vi "JKISM++ Convert Data to HexStr.vi"(2 "Variant":variant) -> (7 "HEX String (0-9,A-F)":string)   [LabVIEW 2014, in "JKI State Machine++.lvlib"]
doc: "Convert complex argument(variant) to hex string, which could be safely used as state argument without broking the string queue logic.\n\n<b>Inputs:</b>\n - <b>Variant</b>: Complex data in variant format.\n\n<b>Outputs:</b>\n - <b>HEX String (0-9,A-F)</b>: Hex String, which contains no invisible string following JKISM's rule"
uses:
  JKI State Machine++.lvlib
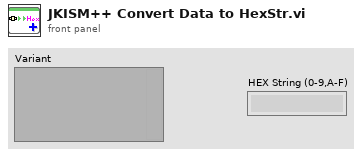
[diagram p1: front panel]
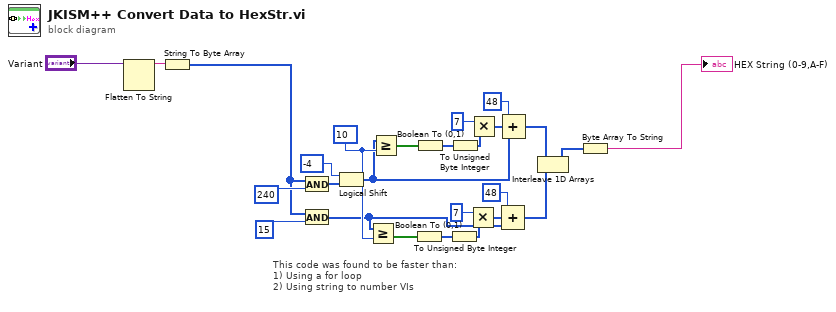
[diagram p0: block diagram]
diagram:
  w20 = u8 10
  # "This code was found to be faster than:\n1) Using a for loop\n2) Using string to number VIs"
  n1 = Flatten To String(anything="Variant") -> (data string=w25:string)  [unwired: 3 in, 2 out]
  n2 = String To Byte Array(string=w25) -> (unsigned byte array=w1:u8[])
  n3 = And(x=w1, y=u8 240) -> (x .and. y?=w22:u8[])
  n4 = And(x=w1, y=u8 15) -> (x .and. y?=w4:u8[])
  n5 = Logical Shift(y=i8 -4, x=w22) -> (x << y=w13:u8[])
  n6 = Greater Or Equal?(x=w4, y=w20) -> (x >= y?=w5:bool[])
  n7 = Greater Or Equal?(x=w13, y=w20) -> (x >= y?=w14:bool[])
  n8 = Boolean To (0,1)(Boolean=w5) -> (0, 1=w7:i16[])
  n9 = Boolean To (0,1)(Boolean=w14) -> (0, 1=w19:i16[])
  n10 = To Unsigned Byte Integer(number=w7) -> (unsigned 8bit integer=w8:u8[])
  n11 = To Unsigned Byte Integer(number=w19) -> (unsigned 8bit integer=w18:u8[])
  n12 = Multiply(x=u8 7, y=w8) -> (x*y=w10:u8[])
  n13 = Multiply(x=u8 7, y=w18) -> (x*y=w16:u8[])
  n14 = Compound Arithmetic op=ADD(u8 48, w10, w4) -> (w3:u8[])
  n15 = Compound Arithmetic op=ADD(u8 48, w16, w13) -> (w12:u8[])
  n16 = Interleave 1D Arrays(w12, w3) -> (w11:u8[])
  n17 = Byte Array To String(unsigned byte array=w11) -> (string=→"HEX String (0-9,A-F)":string)
